vi "Set Topic Attribute.vi"(8 "error in (no error)":errorcluster, 10 "Topic Attribute":T1, 11 "Topic":refnum<class "Topic.lvclass">) -> (0 "error out":errorcluster, 3 "Topic out":refnum<class "Topic.lvclass">)   [LabVIEW 2015, in "NI_AWS_SNS.lvlib" / "Topic.lvclass"]
uses:
  Topic.lvclass
  Mutable Topic Attribute Value Pair.ctl
  Mutable Topic Attribute.ctl
  Core/HTTP Request/Request Options.ctl
  Core/HTTP Request/Name Value Pair.ctl
  Core/ARN/ARN.lvclass/ARN.ctl
  Core/ARN/Read ARN.vi
  Core/HTTP Request/HTTP Request.lvclass
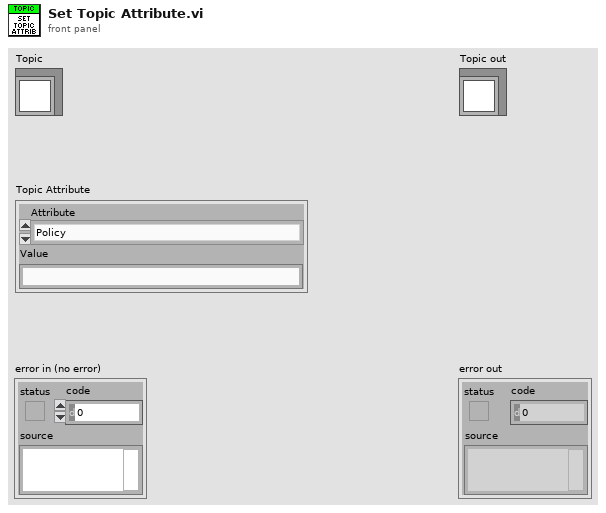
[diagram p1: front panel]
types:
  T1 = typedef "NI_AWS_SNS.lvlib/Topic.lvclass/Mutable Topic Attribute Value Pair.ctl" = cluster{"Attribute":T2, "Value":string}
  T2 = typedef "NI_AWS_SNS.lvlib/Topic.lvclass/Mutable Topic Attribute.ctl" = enum16{"Policy", "DisplayName", "DeliveryPolicy"}
  T3 = typedef "NI_AWS_Core.lvlib/HTTP Request.lvclass/Name Value Pair.ctl" = cluster{"name":string, "value":string}
  T4 = typedef "NI_AWS_Core.lvlib/HTTP Request.lvclass/Request Options.ctl" = cluster{"request headers":T3[], "request parameters":T3[], "request body":string}
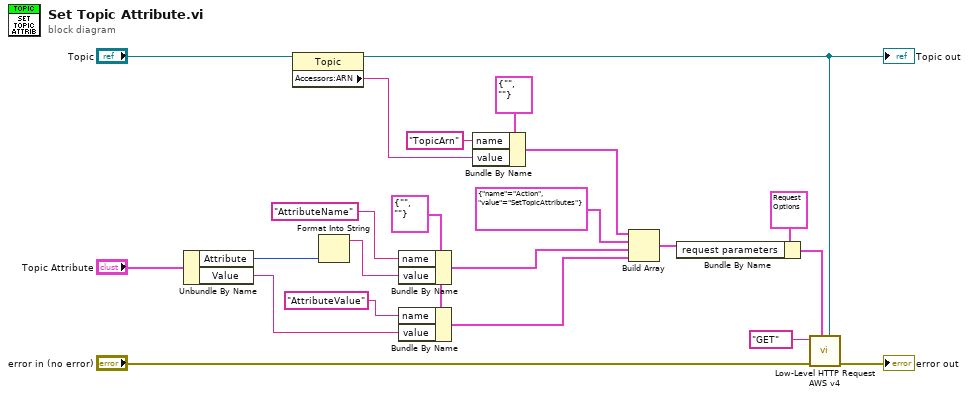
[diagram p0: block diagram]
diagram:
  w3 = T3 {"name"="", "value"=""} ("element")
  n1 = Unbundle By Name("Topic Attribute") -> ("Attribute"=w6:T2, "Value"=w1:string)
  n2 = property class="Topic"(reference="Topic") -> (reference out=w15:refnum<class "Topic.lvclass">, "Accessors:ARN"=w8:string)  [unwired: 1 in, 1 out]
  "Topic out" <- w15
  n3 = Format Into String(w6) -> (resulting string=w4:string)  [unwired: 3 in, 1 out]
  n4 = Bundle By Name(cluster=w3, "name"="AttributeName", "value"=w4) -> (w12:T3)
  n5 = Bundle By Name(cluster=w3, "name"="AttributeValue", "value"=w1) -> (w11:T3)
  n6 = Bundle By Name(cluster=T3 {"name"="", "value"=""} ("element"), "name"="TopicArn", "value"=w8) -> (w7:T3)
  n7 = Build Array(w7, T3 {"name"="Action", "value"="SetTopicAttributes"} ("Cluster"), w12, w11) -> (w13:T3[])
  n8 = Bundle By Name(cluster=T4 {"request headers"=[], "request parameters"=[{"name"="Action", "value"="ListQueues"}], "request body"=""} ("Request Options"), "request parameters"=w13) -> (w16:T4)
  n9 = call "Low-Level HTTP Request AWS v4.vi"("AWS Core"=w15, "Request Options"=w16, "error in (no error)"="error in (no error)", "HTTP-Verb"="GET") -> ("error out"=→"error out":errorcluster)  [unwired: 5 in, 2 out]
